vi "niRFUtil WFM Align Waveforms - Fine (complex wfm).vi"(0 "Waveform In":T2 {"y" format="%.2f"; "dx" format="%^.2e"; "x0" format="%^.2e"}, 5 "Reference Waveform":T2 {"y" format="%.2f"; "dx" format="%^.2e"; "x0" format="%^.2e"}, 7 "Filter Phase Estimates":T1=enum."True", 9 "Filter Length (samples)":i32=20, 11 "error in (no error)":errorcluster, 13 "Flush Buffers?":bool) -> (4 "Waveform Out":T2 {"y" format="%.2f"; "dx" format="%^.2e"; "x0" format="%^.2e"}, 15 "error out":errorcluster)   [LabVIEW 2015, in "niRFUtil.lvlib"]
doc: "(c) Copyright 2006, National Instruments, Inc. This VI may not be duplicated, sold, or distributed without written consent from National Instruments."
uses:
  niRFUtil.lvlib
  Includes/niRFUtil INC Complex Waveform.ctl
  Includes/niRFUtil INC Complex Array.ctl
  Includes/niRFUtil INC Filter Phase Estimates.ctl
  niRFUtil WFM Moving Average (complex array).vi
  Filters, Transforms, Windows/niRFUtil FTW FFT (complex wfm).vi
  niRFUtil WFM Complex Differential (complex wfm).vi
  niRFUtil WFM Parse Waveform - Duration (complex wfm).vi
  Measurements/niRFUtil MEAS Waveform Statistics (complex wfm).vi
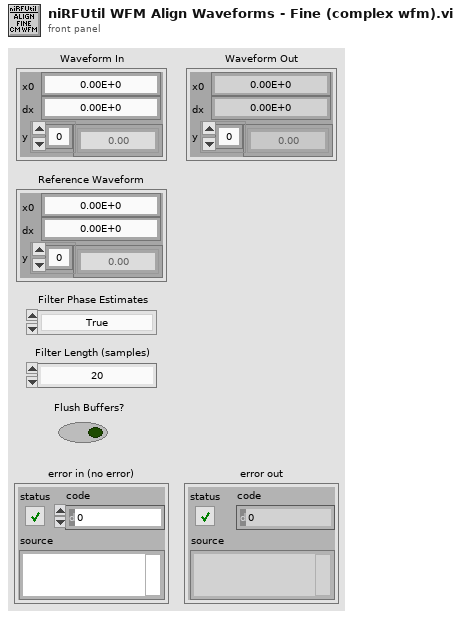
[diagram p1: front panel]
types:
  T1 = typedef "niRFUtil.lvlib/niRFUtil INC Filter Phase Estimates.ctl" = enum16{"False", "True"}
  T2 = typedef "niRFUtil.lvlib/niRFUtil INC Complex Waveform.ctl" = cluster{"x0":dbl, "dx":dbl, "y":T3}
  T3 = typedef "niRFUtil.lvlib/niRFUtil INC Complex Array.ctl" = csg[]
  T4 = typedef "niRFUtil.lvlib/niRFUtil INC Real Array.ctl" = sgl[]
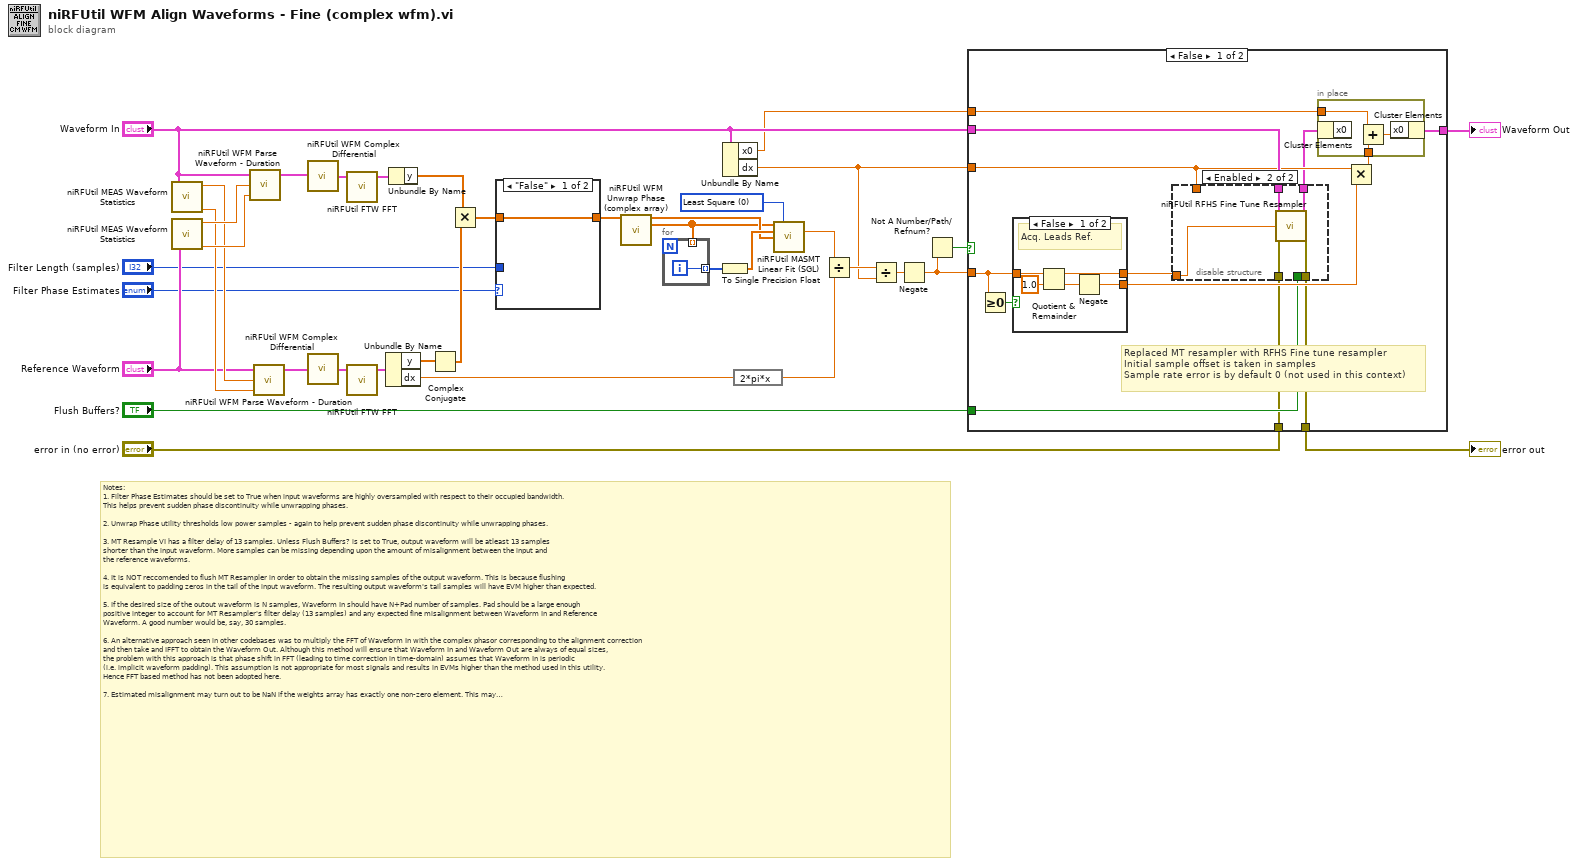
[diagram p0: block diagram]
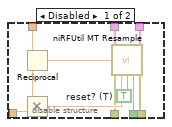
[diagram p2: hidden frame]
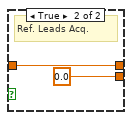
[diagram p3: hidden frame]
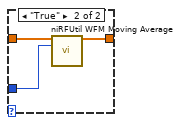
[diagram p5: hidden frame]
diagram:
  w28 = 0 items=["Least Square", "Least Absolute Residual", "Bisquare"] ("method")
  # "Notes:\n1. Filter Phase Estimates should be set to True when input waveforms are highly oversampled with respect to their occupied bandwidth. \nThis helps prevent sudden phase discontinuity while unwrapping phases.\n\n2. Unwrap Phase utility thresholds low power samples - again to help prevent sudden phase discontinuity while unwrapping phases.\n\n3. MT Resample VI has a filter delay of 13 samples. Unless Flush Buffers? is set to True, output waveform will be atleast 13 samples \nshorter than the input waveform. More samples can be missing depending upon the amount of misalignment between the input and\nthe reference waveforms.\n\n4. It is NOT reccomended to flush MT Resampler in order to obtain the missing samples of the output waveform. This is because flushing\nis equivalent to padding zeros in the tail of the input waveform. The resulting output waveform's tail samples will have EVM higher than expected.\n\n5. If the desired size of the outout waveform is N samples, Waveform In should have N+Pad number of samples. Pad should be a large enough \npositive integer to account for MT Resampler's filter delay (13 samples) and any expected fine misalignment between Waveform In and Reference\nWaveform. A good number would be, say, 30 samples.\n\n6. An alternative approach seen in other codebases was to multiply the FFT of Waveform In with the complex phasor corresponding to the alignment correction\nand then take and IFFT to obtain the Waveform Out. Although this method will ensure that Waveform In and Waveform Out are always of equal sizes,\nthe problem with this approach is that phase shift in FFT (leading to time correction in time-domain) assumes that Waveform In is periodic \n(i.e. implicit waveform padding). This assumption is not appropriate for most signals and results in EVMs higher than the method used in this utility.\nHence FFT based method has not been adopted here.\n\n7. Estimated misalignment may turn out to be NaN if the weights array has exactly one non-zero element. This may happen with sinusoids. \nIn that case, no correction is done."
  n1 = call-poly "niRFUtil MEAS Waveform Statistics.vi"("Waveform In"="Waveform In") -> ("Start"=w21:dbl, "Duration"=w22:dbl)  [unwired: 6 out]
  n2 = call-poly "niRFUtil MEAS Waveform Statistics.vi"("Waveform In"="Reference Waveform") -> ("Start"=w23:dbl, "Duration"=w24:dbl)  [unwired: 6 out]
  n3 = call-poly "niRFUtil WFM Parse Waveform - Duration.vi"("Duration (Inf)"=w24, "Start (-Inf)"=w23, "Waveform In"="Waveform In") -> ("Waveform Out"=w27:T2)  [unwired: 2 out]
  n4 = call-poly "niRFUtil WFM Parse Waveform - Duration.vi"("Duration (Inf)"=w22, "Start (-Inf)"=w21, "Waveform In"="Reference Waveform") -> ("Waveform Out"=w25:T2)  [unwired: 2 out]
  n5 = call-poly "niRFUtil WFM Complex Differential.vi"("Waveform In"=w27) -> ("Waveform Out"=w30:T2)  [unwired: 14 out]
  n6 = call-poly "niRFUtil WFM Complex Differential.vi"("Waveform In"=w25) -> ("Waveform Out"=w37:T2)  [unwired: 14 out]
  n7 = call-poly "niRFUtil FTW FFT.vi"("Waveform In (V)"=w30) -> ("Waveform Out (V)"=w16:T2)  [unwired: 2 in, 2 out]
  n8 = call-poly "niRFUtil FTW FFT.vi"("Waveform In (V)"=w37) -> ("Waveform Out (V)"=w15:T2)  [unwired: 2 in, 2 out]
  n9 = Unbundle By Name(w15) -> ("y"=w13:T3, "dx"=w35:dbl)
  n10 = Unbundle By Name(w16) -> ("y"=w14:T3)
  n11 = Complex Conjugate(1:w13) -> (0:w19:T3)
  n12 = Multiply(x=w14, y=w19) -> (x*y=w17:T3)
  n13 = case shown="\"False\"" "Filter Phase Estimates" {
    tunnel: w17 -> [w38 w41]
    tunnel: [w38 w40] -> w12
    tunnel: "Filter Length (samples)" -> [_ w39]
    frame "False" {
    }
    frame "True" {
      n14 = call-poly "niRFUtil WFM Moving Average.vi"("Array In"=w41, "Averaging Window (samples)"=w39) -> ("Averaged Array Out"=w40:T3)  [unwired: 13 in]
    }
  }
  n15 = call "niRFUtil WFM Unwrap Phase (complex array).vi"("Complex Vectors"=w12) -> ("Magnitude"=w11:T4, "Unwrapped Phase (rad)"=w10:T4)  [unwired: 13 in]
  n16 = for {
    tunnel: [w42] -> w36 mode=indexing
    tunnel: w10 -> [_] mode=indexing
    i -> [w42]
  }
  n17 = To Single Precision Float(number=w36) -> (single precision float=w18:sgl[])
  n18 = Unbundle By Name("Waveform In") -> ("x0"=w3:dbl, "dx"=w4:dbl)
  n19 = expression code="2*pi*x"(w35) -> (w33:dbl)
  n20 = call "niRFUtil MASMT Linear Fit (SGL).vi"("Y"=w10, "method"=w28, "X"=w18, "Weight"=w11) -> ("slope"=w34:sgl)  [unwired: 7 in, 4 out]
  n21 = Divide(x=w34, y=w33) -> (x/y=w32:dbl)
  n22 = Divide(x=w32, y=w4) -> (x/y=w31:dbl)
  n23 = Negate(x=w31) -> (-x=w6:dbl)
  n24 = Not A Number/Path/Refnum?(number/path/refnum=w6) -> (NaN/Path/Refnum?=w7:bool)
  n25 = case shown="False" w7 {
    tunnel: w6 -> [w49 _]
    tunnel: [w55 w82] -> w29
    tunnel: "Waveform In" -> [w54 w82]
    tunnel: "Flush Buffers?" -> [w51 _]
    tunnel: w4 -> [w50 _]
    tunnel: w3 -> [w48 _]
    tunnel: "error in (no error)" -> [w44 w81]
    tunnel: [w43 w81] -> w1
    frame False {
      # "Replaced MT resampler with RFHS Fine tune resampler\nInitial sample offset is taken in samples\nSample rate error is by default 0 (not used in this context)"
      n26 = Greater Or Equal To 0?(x=w49) -> (x >= 0?=w53:bool)
      n27 = case shown="False" w53 {
        tunnel: [w74 0.0] -> w52
        tunnel: w49 -> [w78 w80]
        tunnel: [w75 w80] -> w45
        frame False {
          # "Acq. Leads Ref."
          n28 = Quotient & Remainder(x=w78, y=1.0) -> (x-y*floor(x/y)=w75:dbl, floor(x/y)=w76:dbl)
          n29 = Negate(x=w76) -> (-x=w74:dbl)
        }
        frame True {
          # "Ref. Leads Acq."
        }
      }
      n30 = disable-structure shown="Enabled" {
        disable-tunnel: w54 -> [w65 w70]
        disable-tunnel: w51 -> [w64 _]
        disable-tunnel: w50 -> [w63 _]
        disable-tunnel: [w60 w69] -> w47
        disable-tunnel: w45 -> [w58 w68]
        disable-tunnel: w44 -> [w57 w67]
        disable-tunnel: [w56 w66] -> w43
        frame Disabled {
          w62 = TRUE  # reset? (T)
          n31 = Reciprocal(x=w63) -> (1/x=w61:dbl)
          n32 = Multiply(x=w63, y=w58) -> (x*y=w59:dbl)
          n33 = call "niRFUtil MT Resample.vi"("Waveform In"=w65, "initial sample offset (sec)"=w59, "desired sample rate (Hz)"=w61, "error in (no error)"=w57, "reset? (T)"=w62, "flush buffers? (F)"=w64) -> ("Waveform Out"=w60:T2, "error out"=w56:errorcluster)  [unwired: 8 in]
        }
        frame Enabled {
          n34 = call "niRFUtil RFHS Fine Tune Resampler.vi"("Complex Waveform In"=w70, "Initial Sample Offset (samples)"=w68, "error in (no error)"=w67) -> ("Complex Waveform Out"=w69:T2, "error out"=w66:errorcluster)  [unwired: 11 in]
        }
      }
      n35 = Multiply(x=w50, y=w52) -> (x*y=w46:dbl)
      n36 = in-place {
        in-place-border: w46 -> [w72]
        in-place-border: w48 -> [w71]
        n37 = in-place-cluster #1(w47) -> ()  [unwired: 1 out]
        n38 = Add(x=w71, y=w72) -> (x+y=w73:dbl)
        n39 = in-place-cluster #1("x0"=w73) -> (w55:T2)
      }
    }
    frame True {
    }
  }
  "Waveform Out" <- w29
  "error out" <- w1
